vi "worksheet set top left cell.vi"(8 "error in (no error)":errorcluster, 9 "col":u16, 10 "row":u32, 11 "worksheet":u32) -> (0 "error out":errorcluster)   [LabVIEW 8.6]
doc: "void worksheet_set_top_left_cell(lxw_worksheet worksheet, lxw_row_t row, lxw_col_t col);"
uses:
  pending_lvxlsxwriter/xlsxwriter.dll
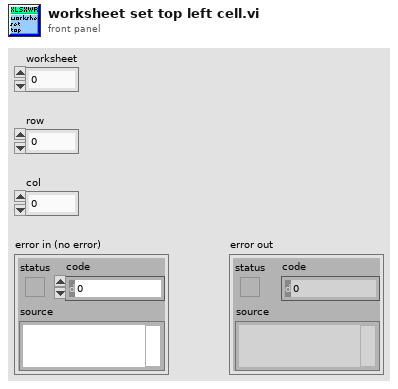
[diagram p1: front panel]
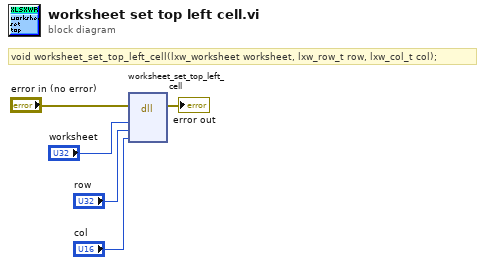
[diagram p0: block diagram]
diagram:
  # "void worksheet_set_top_left_cell(lxw_worksheet worksheet, lxw_row_t row, lxw_col_t col);"
  n1 = dll-call lib="C:/Users/WDAGUtilityAccount/Desktop/pending_lvxlsxwriter/xlsxwriter.*" fn="worksheet_set_top_left_cell"(error in="error in (no error)", "worksheet"="worksheet", "row"="row", "col"="col") -> (error out=→"error out":errorcluster)  [unwired: 6 in, 1 out]
